vi "CHD_SIM_Motor_Write.vi"(10 "Motor Demand":dbl, 11 "Motor Device Reference":T1={"DeviceStatus"={"status"=FALSE, "code"=0, "source"=""}, "Type"=enum."PWM", "PWM"={"PWM Channel"=enum."Invalid", "DeadBand"={"Name"="", "maxPositivePwm"=0, "minPositivePwm"=0, "centerPwm"=0, "maxNegativePwm"=0, "minNegativePwm"=0, "angularRange"=0}}, "CAN"={"Device Number"=0, "SetOutput VI Ref"=variant, "GetOutput VI Ref"=variant, "Enable VI Ref"=variant, "Disable VI Ref"=variant, "Data"=variant}, "Invert"=FALSE, "DIO PWM"={"PWM \"Enable\" Channel"=enum."Invalid", "DIOChannel"=enum."Invalid", "PWM Rate"=0.0}}) -> (3 "Out Motor Demand":dbl)   [LabVIEW 2019]
uses:
  <vilib>/Rock Robotics/WPI/MotorControl/WPI_MotorControlDeviceRef.ctl
  <vilib>/Rock Robotics/WPI/MotorControl/WPI_MotorControlType.ctl
  <vilib>/Rock Robotics/SystemInterfaces/DIO/FPGA_DIOPWMChannel.ctl
  <vilib>/Rock Robotics/WPI/PWM/WPI_PWMDeadband.ctl
  <vilib>/Rock Robotics/SystemInterfaces/DIO/FPGA_DIOChannel.ctl
  CHD_SIM_SIM_Globals.vi
  <vilib>/Rock Robotics/WPI/ThirdParty/JAS_Junk/TrajLib/Trajectory_Library.lvlib
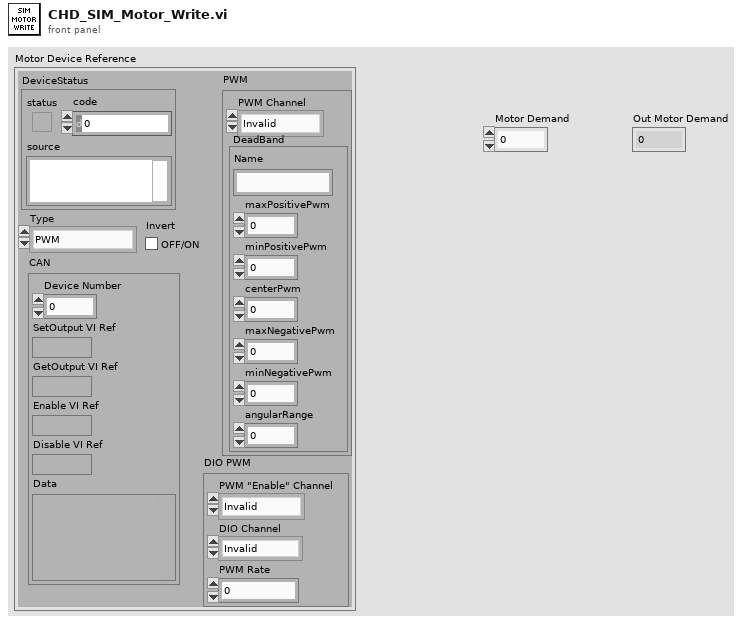
[diagram p1: front panel]
types:
  T1 = typedef "WPI_MotorControlDeviceRef.ctl" = cluster{"DeviceStatus":errorcluster, "Type":T2, "PWM":cluster{"PWM Channel":T3, "DeadBand":T4}, "CAN":cluster{"Device Number":u8, "SetOutput VI Ref":variant, "GetOutput VI Ref":variant, "Enable VI Ref":variant, "Disable VI Ref":variant, "Data":variant}, "Invert":bool, "DIO PWM":cluster{"PWM \"Enable\" Channel":T3, "DIOChannel":T5, "PWM Rate":dbl}}
  T2 = typedef "WPI_MotorControlType.ctl" = enum16{"PWM", "CAN", "DIO PWM"}
  T3 = typedef "FPGA_DIOPWMChannel.ctl" = enum8{"PWM 0", "PWM 1", "PWM 2", "PWM 3", "PWM 4", "PWM 5", "PWM 6", "PWM 7", "PWM 8", "PWM 9", "PWM MXP 0", "PWM MXP 1", "PWM MXP 2", "PWM MXP 3", "PWM MXP 4", "PWM MXP 5", "PWM MXP 6", "PWM MXP 7", "PWM MXP 8", "PWM MXP 9", "Invalid"}
  T4 = typedef "WPI_PWMDeadband.ctl" = cluster{"Name":string, "maxPositivePwm":i32, "minPositivePwm":i32, "centerPwm":i32, "maxNegativePwm":i32, "minNegativePwm":i32, "angularRange":u16}
  T5 = typedef "FPGA_DIOChannel.ctl" = enum8{"DIO 0", "DIO 1", "DIO 2", "DIO 3", "DIO 4", "DIO 5", "DIO 6", "DIO 7", "DIO 8", "DIO 9", "DIO MXP 0", "DIO MXP 1", "DIO MXP 2", "DIO MXP 3", "DIO MXP 4", "DIO MXP 5", "DIO MXP 6", "DIO MXP 7", "DIO MXP 8", "DIO MXP 9", "DIO MXP 10", "DIO MXP 11", "DIO MXP 12", "DIO MXP 13", "DIO MXP 14", "DIO MXP 15", "SPI Port CS1", "SPI Port CS2", "SPI Port CS3", "SPI Port MISO", "SPI Port MOSI", "Invalid"}
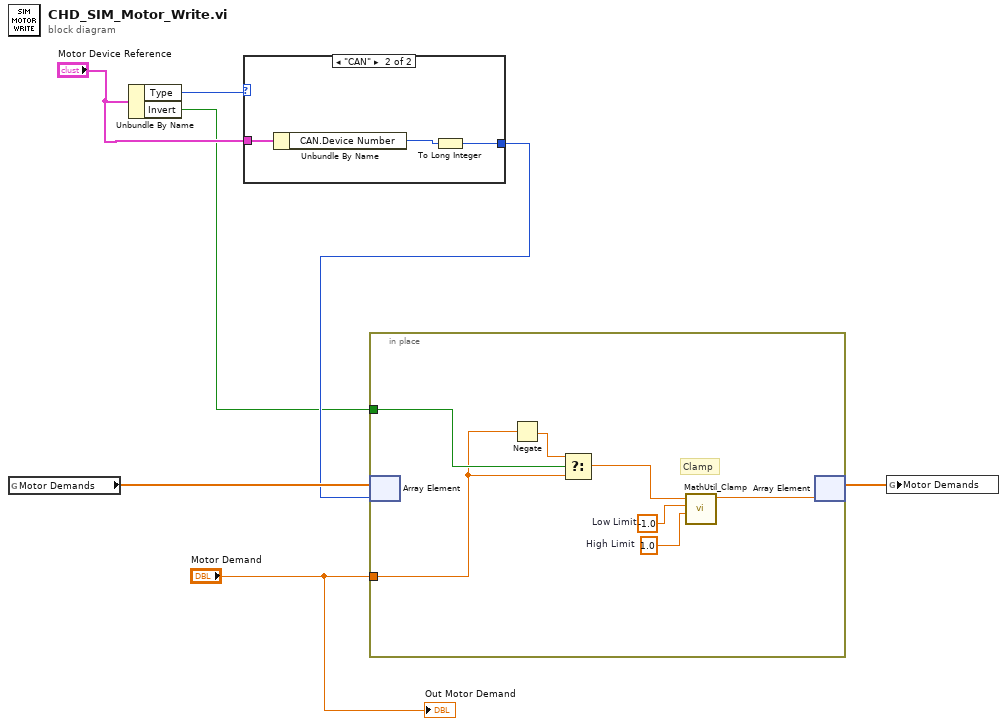
[diagram p0: block diagram]
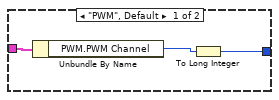
[diagram p2: hidden frame]
diagram:
  n1 = global read "CHD_SIM_SIM_Globals.vi" "Motor Demands"() -> (w7:dbl[])
  n2 = Unbundle By Name("Motor Device Reference") -> ("Type"=w6:T2, "Invert"=w1:bool)
  n3 = case shown="\"CAN\"" w6 {
    tunnel: "Motor Device Reference" -> [w10 w12]
    tunnel: [w8 w11] -> w4
    frame "PWM", Default {
      n4 = Unbundle By Name(w10) -> ("PWM.PWM Channel"=w9:T3)
      n5 = To Long Integer(number=w9) -> (32bit integer=w8:i32)
    }
    frame "CAN" {
      n6 = Unbundle By Name(w12) -> ("CAN.Device Number"=w13:u8)
      n7 = To Long Integer(number=w13) -> (32bit integer=w11:i32)
    }
  }
  n8 = in-place {
    in-place-border: "Motor Demand" -> [w16]
    in-place-border: w1 -> [w17]
    w20 = 1.0  # High Limit
    w19 = -1.0  # Low Limit
    # "Clamp"
    n9 = in-place-array #1(w7, w4) -> ()  [unwired: 1 out]
    n10 = Negate(x=w16) -> (-x=w15:dbl)
    n11 = Select(t=w15, s=w17, f=w16) -> (s? t:f=w14:dbl)
    n12 = call <vilib>:"MathUtil_Clamp.vi"("High Limit"=w20, "Low Limit"=w19, "Value"=w14) -> ("Result"=w18:dbl)  [unwired: 8 in]
    n13 = in-place-array #1(w18) -> (w3:dbl[])  [unwired: 1 out]
  }
  n14 = global write "CHD_SIM_SIM_Globals.vi" "Motor Demands"(w3) -> ()
  "Out Motor Demand" <- "Motor Demand"
